vi "BinaryInvert.vi"(3 "Image In":T1 {"Dialogs" format="%.0b"}) -> (1 "Image Out":T1 {"Dialogs" format="%.0b"})   [LabVIEW 2024]
doc: "This VI will invert a 1 bit image. All ones will be zeros and vice versa."
uses:
  <userlib>/ImageProcessing/QTLIB_2595_LV86/QT_Image.ctl
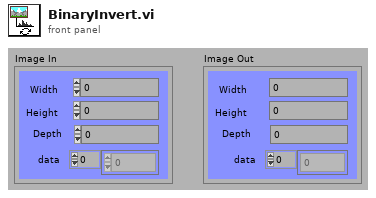
[diagram p1: front panel]
types:
  T1 = typedef "QT_Image.ctl" = cluster{"Width":i32, "Height":i32, "Depth":i32, "data":u8[], "Compressed data":u8[], "Color table":u32[], "Duration":i32, "Options":i32, "Timestamp":i32, "ID":i32, "Reserved":i32, "Dialogs":u32}
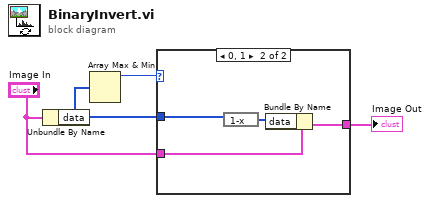
[diagram p0: block diagram]
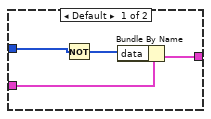
[diagram p2: hidden frame]
diagram:
  n1 = Unbundle By Name("Image In") -> ("data"=w2:u8[])
  n2 = Array Max & Min(array=w2) -> (max value=w1:u8)  [unwired: 3 out]
  n3 = case shown="0, 1" w1 {
    tunnel: [w8 w12] -> w4
    tunnel: w2 -> [w6 w9]
    tunnel: "Image In" -> [w7 w10]
    frame Default {
      n4 = Not(x=w6) -> (.not. x?=w5:u8[])
      n5 = Bundle By Name(cluster=w7, "data"=w5) -> (w8:T1)
    }
    frame 0, 1 {
      n6 = expression code="1-x"(w9) -> (w11:u8[])
      n7 = Bundle By Name(cluster=w10, "data"=w11) -> (w12:T1)
    }
  }
  "Image Out" <- w4
